vi "Get optimal sampling rate.vi"(10 "sweep time":dbl) -> (1 "sample rate index":i32, 2 "sampl rate":dbl)   [LabVIEW 2017]
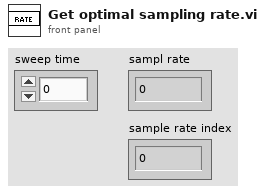
[diagram p1: front panel]
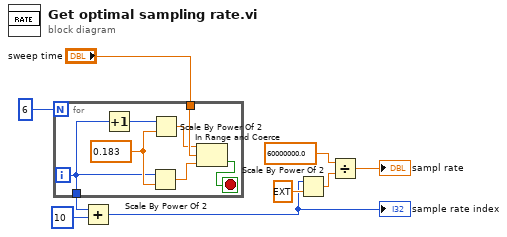
[diagram p0: block diagram]
diagram:
  n1 = for {
    N: 6 -> [_]
    tunnel: "sweep time" -> [w16]
    tunnel: [w10] -> w2
    i -> [w10]
    stop <- w15 stop-if-true
    w13 = 0.183
    n2 = Increment(x=w10) -> (x+1=w14:i32)
    n3 = Scale By Power Of 2(n=w10, x=w13) -> (x*2^n=w11:dbl)
    n4 = Scale By Power Of 2(n=w14, x=w13) -> (x*2^n=w12:dbl)
    n5 = In Range and Coerce(upper limit=w12, x=w16, lower limit=w11) -> (In Range?=w15:bool)  [unwired: 1 out]
  }
  n6 = Add(x=w2, y=10) -> (x+y=w5:i32)
  "sample rate index" <- w5
  n7 = Scale By Power Of 2(n=w5, x=ext 1.0) -> (x*2^n=w6:ext)
  n8 = Divide(x=60000000.0, y=w6) -> (x/y=→"sampl rate":ext)
